vi "Choose Serial port.vi"(2 "Path":path, 3 "Current Serial Port Aliases":string[][](array[string]), 4 "Message":string) -> (1 "Choosen Port":string)   [LabVIEW 2022 SP3]
uses:
  <vilib>/Instr/_visa.llb/VISA Find Search Mode.ctl
panel:
  out "File Path if you need to edit these  values":path
  out "Serial Port Aliases Out":string[][](array[string])
  in  "stop":bool
  in  "OK":bool
  in  "Selector":i32[](listbox)
  in  "Refresh Port List":bool
  out "Previous  List":string[](array[string])
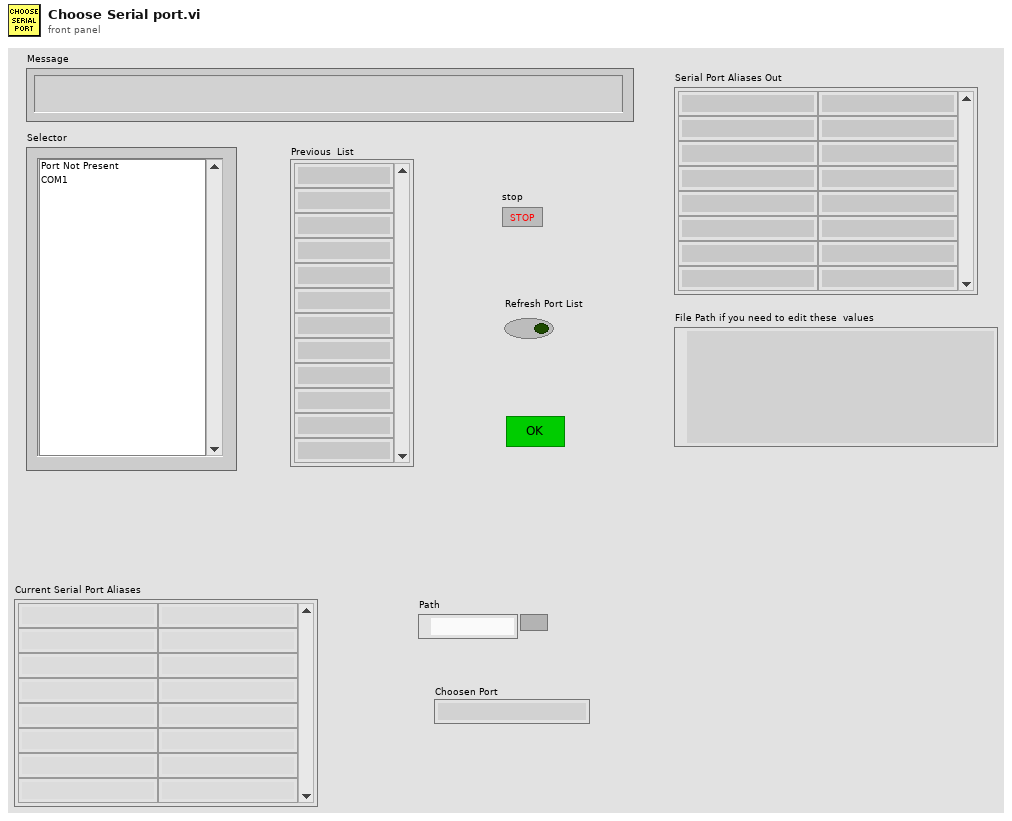
[diagram p1: front panel]
types:
  T1 = typedef "VISA Find Search Mode.ctl" = u32
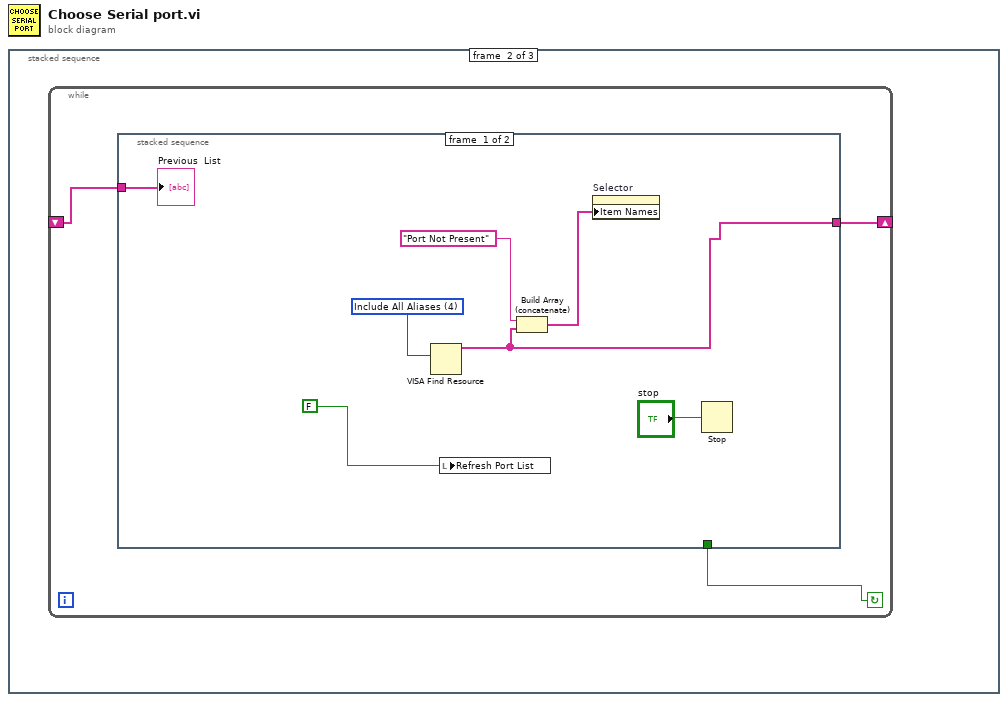
[diagram p0: block diagram]
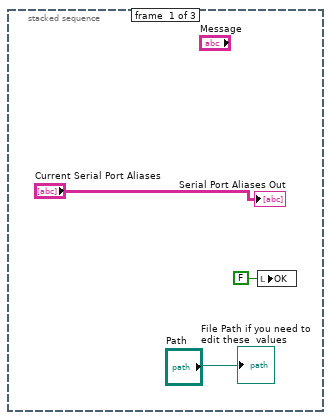
[diagram p2: hidden frame]
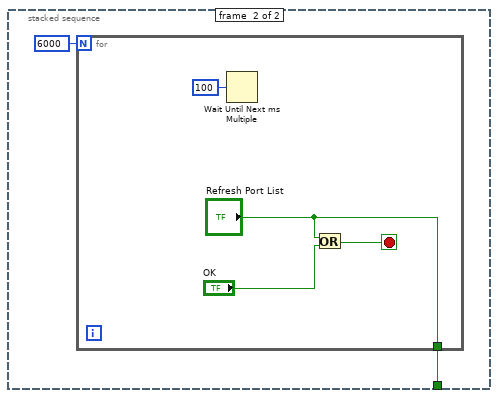
[diagram p3: hidden frame]
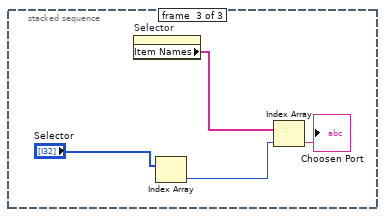
[diagram p4: hidden frame]
diagram:
  n1 = stacked-sequence {
    frame #0 {
      n2 = local write "OK"(FALSE ("OK")) -> ()
      "Serial Port Aliases Out" <- "Current Serial Port Aliases"
      "File Path if you need to edit these  values" <- "Path"
    }
    frame #1 {
      n3 = while {
        shift-right: [w5] -> _
        shift-left: _ -> [w6]
        stop <- w4 continue-if-true
        n4 = stacked-sequence {
          tunnel: w6 -> [w12 _]
          tunnel: [w8 _] -> w5
          tunnel: [_ w15] -> w4
          frame #0 {
            w13 = T1 4 items=["Canonical Names Only"=0, "Aliases Only"=1, "Include Matching Aliases"=2, "Include All Aliases"=4] ("Search Mode")
            n5 = VISA Find Resource(10:w13) -> (3:w8:string[])  [unwired: 2 in, 2 out]
            n6 = local write "Refresh Port List"(FALSE ("Refresh List")) -> ()
            n7 = Build Array (concatenate)("Port Not Present", w8) -> (w9:string[])
            n8 = property on="Selector" class="LstBox (strict)"("Item Names"=w9) -> ()  [unwired: 2 in, 2 out]
            n9 = Stop(stop? (T)="stop") -> ()
            "Previous  List" <- w12
          }
          frame #1 {
            n10 = for {
              N: 6000 -> [_]
              tunnel: ["Refresh Port List"] -> w15
              stop <- w16 stop-if-true
              n11 = Wait Until Next ms Multiple(millisecond multiple=u32 100) -> ()  [unwired: 1 out]
              n12 = Or(x="Refresh Port List", y="OK") -> (x .or. y?=w16:bool)
            }
          }
        }
      }
    }
    frame #2 {
      n13 = property on="Selector" class="LstBox (strict)"() -> ("Item Names"=w23:string[])  [unwired: 2 in, 2 out]
      n14 = Index Array(array="Selector") -> (element=w21:i32)  [unwired: 1 in]
      n15 = Index Array(array=w23, index=w21) -> (element=→"Choosen Port":string)
    }
  }
